vi "Perform Power Signals Autosetup.vi"(8 "error in (no error)":errorcluster, 10 "Power Analysis Type (0: Harmonics)":i32(ring) items=["Harmonics", "Efficiency", "Ripple", "Modulation", "Quality", "Slew Rate", "Switch Loss", "RDSVce"], 11 "VISA resource name":refnum<visa-resource-name>) -> (0 "error out":errorcluster, 3 "VISA resource name out":refnum<visa-resource-name>)   [LabVIEW 2015, in "Agilent 2000 3000 X-Series.lvlib"]
doc: "Performs automated oscilloscope setup for the signals in the specified type of power analysis."
uses:
  <instrlib>/Agilent 2000 3000 X-Series/Agilent 2000 3000 X-Series.lvlib
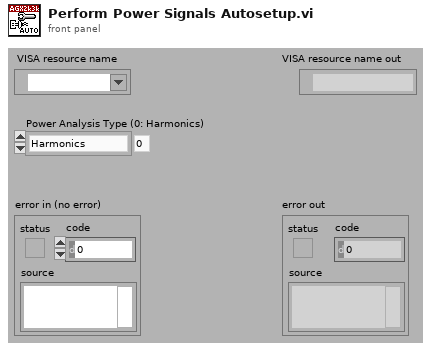
[diagram p1: front panel]
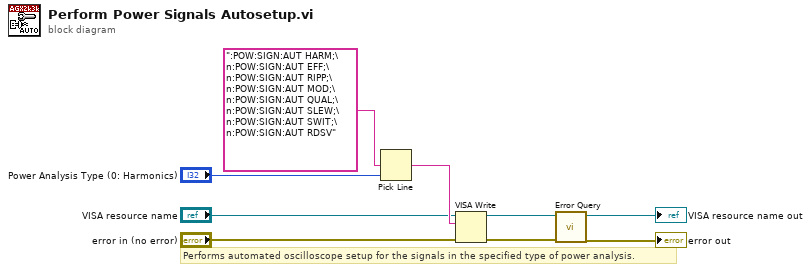
[diagram p0: block diagram]
diagram:
  # "Performs automated oscilloscope setup for the signals in the specified type of power analysis."
  n1 = Pick Line(multi-line string=":POW:SIGN:AUT HARM;\n:POW:SIGN:AUT EFF;\n:POW:SIGN:AUT RIPP;\n:POW:SIGN:AUT MOD;\n:POW:SIGN:AUT QUAL;\n:POW:SIGN:AUT SLEW;\n:POW:SIGN:AUT SWIT;\n:POW:SIGN:AUT RDSV", line index="Power Analysis Type (0: Harmonics)") -> (output string=w7:string)  [unwired: 1 out]
  n2 = VISA Write(VISA resource name="VISA resource name", write buffer=w7, error in (no error)="error in (no error)") -> (VISA resource name out=w4:refnum<visa-resource-name>, error out=w3:errorcluster)  [unwired: 1 out]
  n3 = call <instrlib>:"Error Query.vi"("error in (no error)"=w3, "VISA resource name"=w4) -> ("error out"=→"error out":errorcluster, "VISA resource name out"=→"VISA resource name out":refnum<visa-resource-name>)  [unwired: 8 out]
